vi "Read Source Action.vi"(8 "error in (no error)":errorcluster, 11 "Report Data in":refnum<class "Report Data.lvclass">) -> (0 "error out":errorcluster, 2 "Source Action":refnum<class "Project Action.lvclass">, 3 "Report Data out":refnum<class "Report Data.lvclass">)   [LabVIEW 2019, in "ProjectBuilder.lvlib" / "Report Data.lvclass"]
doc: "Read the source action class from the private data."
uses:
  Report Data.lvclass
  Project Action/Project Action.lvclass
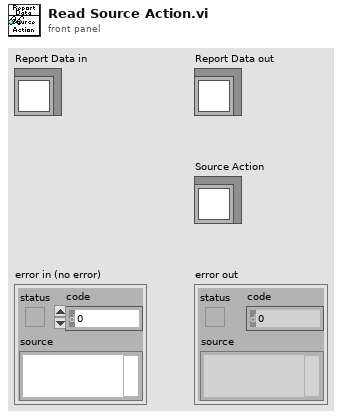
[diagram p1: front panel]
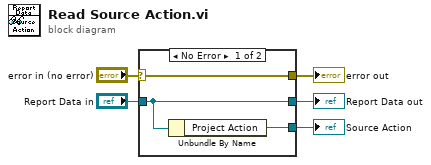
[diagram p0: block diagram]
diagram:
  n1 = case shown="No Error" "error in (no error)" {
    selector: "error in (no error)" -> [w8 w9]
    tunnel: [w8 w9] -> w4
    tunnel: [w7 w10] -> w2
    tunnel: "Report Data in" -> [w7 w10]
    tunnel: [w6 _] -> w1
    frame No Error {
      n2 = Unbundle By Name(w7) -> ("Project Action"=w6:refnum<class "Project Action.lvclass">)
    }
    frame Error {
    }
  }
  "error out" <- w4
  "Report Data out" <- w2
  "Source Action" <- w1
